vi "ReadUSB.vi"() -> ()   [LabVIEW 2017]
uses:
  <vilib>/Instr/_visa.llb/VISA Configure Serial Port (Instr).vi
panel:
  in  "Desired Speed":dbl
  in  "Option":enum16{"Esquerda", "Direita", "Duas rodas"}(ring)
  in  "Write":bool
  in  "End":bool
  out "Vel Wheel D":dbl
  out "String Tratada 2":string
  out "Vel Wheel E":dbl
  out "String Lida":string
  out "config error":errorcluster
  out "String Tratada":string
  out "Vel Wheel Right":cluster{dbl}(graph)
  in  "VISA resource name":refnum<visa-resource-name>
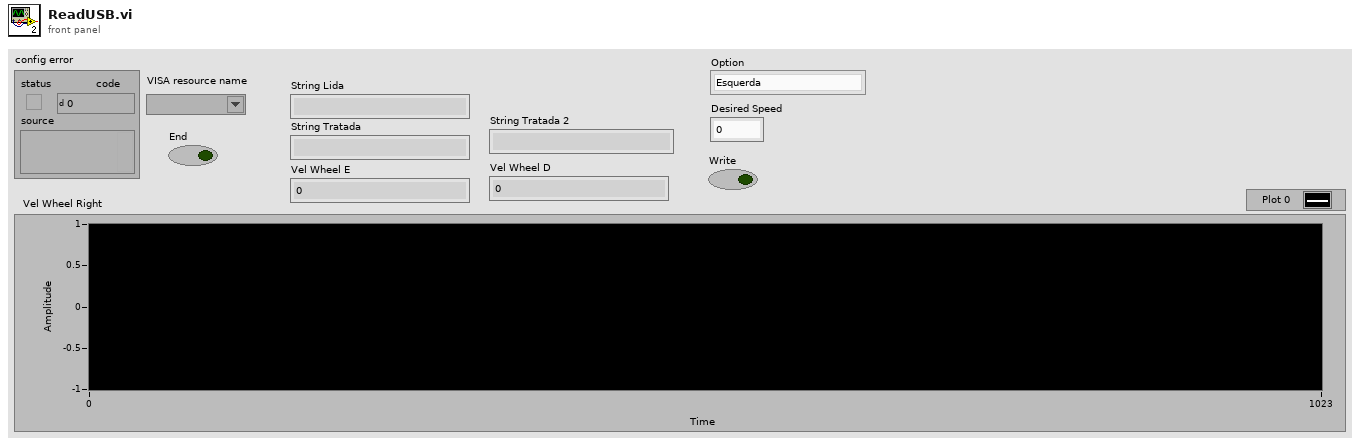
[diagram p1: front panel]
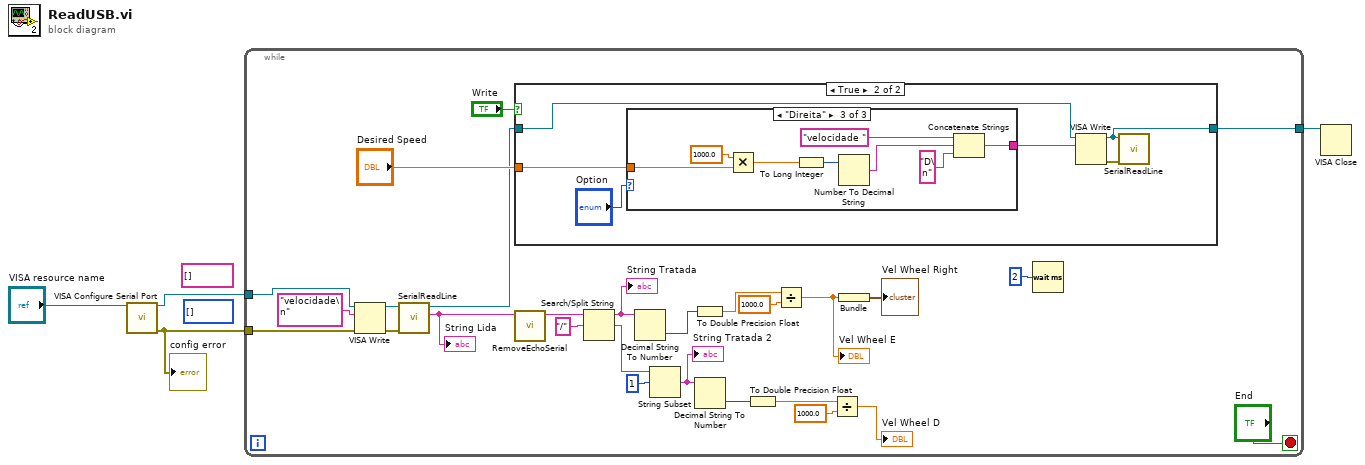
[diagram p0: block diagram]
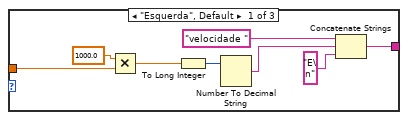
[diagram p3: hidden frame]
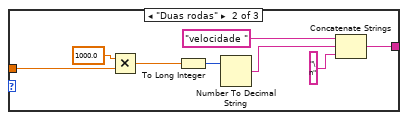
[diagram p4: hidden frame]
diagram:
  (unwired) i32[] []
  (unwired) string[] []
  n1 = call-poly "VISA Configure Serial Port"("VISA resource name"="VISA resource name") -> ("VISA resource name out"=w3:refnum<visa-resource-name>, "error out"=w2:errorcluster)  [unwired: 13 in]
  "config error" <- w2
  n2 = while {
    tunnel: w3 -> [w31]
    tunnel: w2 -> [w30]
    tunnel: [w9] -> w1
    stop <- "End" stop-if-true
    n3 = VISA Write(VISA resource name=w31, write buffer="velocidade\n", error in (no error)=w30) -> (VISA resource name out=w27:refnum<visa-resource-name>, error out=w26:errorcluster)  [unwired: 1 out]
    n4 = call "SerialReadLine.vi"("error in"=w26, "VISA resource name in"=w27) -> ("String"=w22:string, "VISA resource name out"=w10:refnum<visa-resource-name>)  [unwired: 7 in, 1 out]
    "String Lida" <- w22
    n5 = case shown="True" "Write" {
      tunnel: "Desired Speed" -> [_ w37]
      tunnel: w10 -> [w32 w35]
      tunnel: [w32 w34] -> w9
      frame False {
      }
      frame True {
        n6 = case shown="\"Direita\"" "Option" {
          tunnel: w37 -> [w40 w54 w56]
          tunnel: [w39 w47 w55] -> w36
          frame "Esquerda", Default {
            n7 = Multiply(x=1000.0, y=w40) -> (x*y=w45:dbl)
            n8 = To Long Integer(number=w45) -> (32bit integer=w44:i32)
            n9 = Number To Decimal String(number=w44) -> (decimal integer string=w42:string)  [unwired: 1 in]
            n10 = Concatenate Strings("velocidade ", w42, "E\n" ("string")) -> (w39:string)
          }
          frame "Duas rodas" {
            n11 = Multiply(x=1000.0, y=w54) -> (x*y=w52:dbl)
            n12 = To Long Integer(number=w52) -> (32bit integer=w51:i32)
            n13 = Number To Decimal String(number=w51) -> (decimal integer string=w49:string)  [unwired: 1 in]
            n14 = Concatenate Strings("velocidade ", w49, "\n" ("string")) -> (w47:string)
          }
          frame "Direita" {
            n15 = Multiply(x=1000.0, y=w56) -> (x*y=w61:dbl)
            n16 = To Long Integer(number=w61) -> (32bit integer=w60:i32)
            n17 = Number To Decimal String(number=w60) -> (decimal integer string=w58:string)  [unwired: 1 in]
            n18 = Concatenate Strings("velocidade ", w58, "D\n" ("string")) -> (w55:string)
          }
        }
        n19 = VISA Write(VISA resource name=w35, write buffer=w36) -> (VISA resource name out=w34:refnum<visa-resource-name>, error out=w33:errorcluster)  [unwired: 1 in, 1 out]
        n20 = call "SerialReadLine.vi"("error in"=w33, "VISA resource name in"=w34) -> ()  [unwired: 7 in, 3 out]
      }
    }
    n21 = call "RemoveEchoSerial.vi"("String in"=w22) -> ("String out"=w17:string)  [unwired: 10 in]
    n22 = Search/Split String(string=w17, search string/char (-)="/") -> (substring before match=w16:string, match + rest of string=w20:string)  [unwired: 1 in, 1 out]
    "String Tratada" <- w16
    n23 = Decimal String To Number(string=w16) -> (number=w5:i32)  [unwired: 2 in, 1 out]
    n24 = String Subset(string=w20, offset (0)=1) -> (substring=w18:string)  [unwired: 1 in]
    "String Tratada 2" <- w18
    n25 = To Double Precision Float(number=w5) -> (double precision float=w8:dbl)
    n26 = Decimal String To Number(string=w18) -> (number=w7:i32)  [unwired: 2 in, 1 out]
    n27 = To Double Precision Float(number=w7) -> (double precision float=w6:dbl)
    n28 = Divide(x=w8, y=1000.0) -> (x/y=w23:dbl)
    "Vel Wheel E" <- w23
    n29 = Divide(x=w6, y=1000.0) -> (x/y=→"Vel Wheel D":dbl)
    n30 = Bundle(w23) -> (→"Vel Wheel Right":cluster{dbl})  [unwired: 1 in]
    n31 = Wait (ms)(milliseconds to wait=u32 2) -> ()  [unwired: 1 out]
  }
  n32 = VISA Close(VISA resource name=w1) -> ()  [unwired: 1 in, 1 out]
